vi "configure tdms channels.vi"(4 "samples per channel (1)":u16=1, 6 "type order":T2[](array[typedef]), 8 "error in":errorcluster, 9 "dictionary group names":T1, 10 "dictionary":T1, 11 "tdms file in":refnum<k34>) -> (0 "error out":errorcluster, 3 "tdms file out":refnum<k34>)   [LabVIEW 2015, in "TDMS datalogger runtime.lvclass"]
uses:
  TDMS datalogger runtime.lvclass
  <vilib>/NI/Tag Bus/dictionary/full data dictionary.ctl
  <vilib>/NI/Tag Bus/tag/Data Type.ctl
  <vilib>/NI/Tag Bus/tag/tag descriptor.lvclass
  <vilib>/NI/Tag Bus/dictionary/data dictionary.lvclass
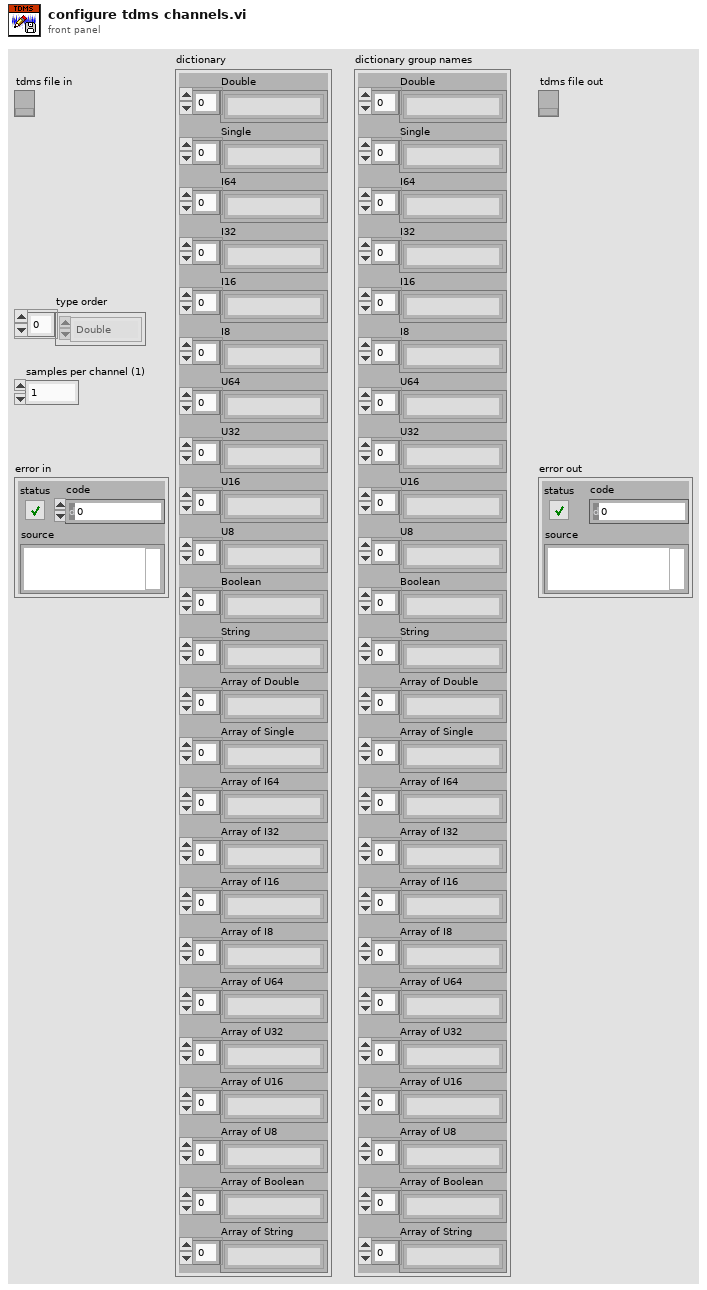
[diagram p1: front panel]
types:
  T1 = typedef "tag bus.lvlib/data dictionary.lvclass/full data dictionary.ctl" = cluster{"Double":string[], "Single":string[], "I64":string[], "I32":string[], "I16":string[], "I8":string[], "U64":string[], "U32":string[], "U16":string[], "U8":string[], "Boolean":string[], "String":string[], "Array of Double":string[], "Array of Single":string[], "Array of I64":string[], "Array of I32":string[], "Array of I16":string[], "Array of I8":string[], "Array of U64":string[], "Array of U32":string[], "Array of U16":string[], "Array of U8":string[], "Array of Boolean":string[], "Array of String":string[]}
  T2 = typedef "tag bus.lvlib/tag descriptor.lvclass/Data Type.ctl" = enum16{"Double", "Single", "I64", "I32", "I16", "I8", "U64", "U32", "U16", "U8", "Boolean", "String", "Array of Double", "Array of Single", "Array of I64", "Array of I32", "Array of I16", "Array of I8", "Array of U64", "Array of U32", "Array of U16", "Array of U8", "Array of Boolean", "Array of String"}
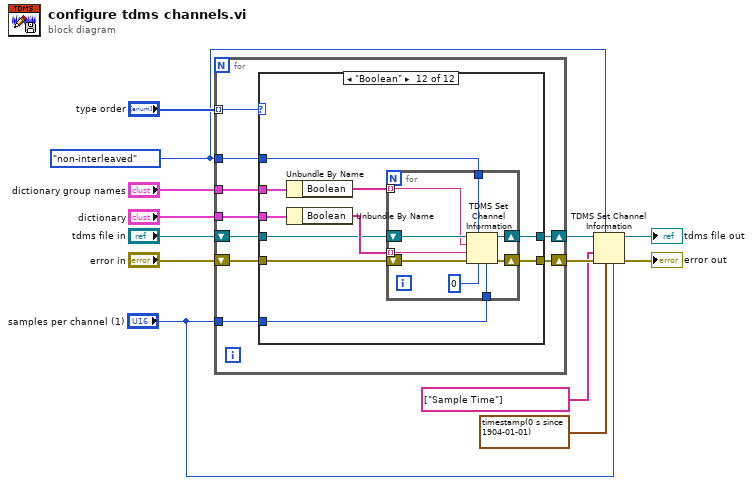
[diagram p0: block diagram]
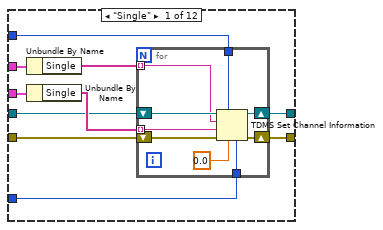
[diagram p2: hidden frame]
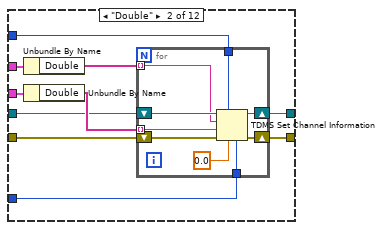
[diagram p3: hidden frame]
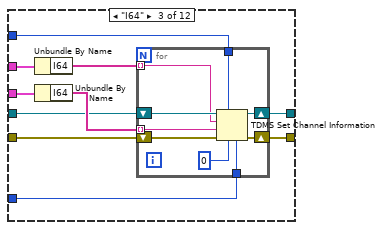
[diagram p4: hidden frame]
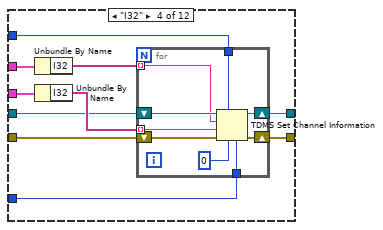
[diagram p5: hidden frame]
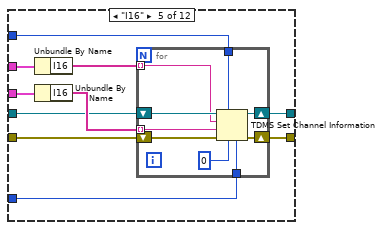
[diagram p6: hidden frame]
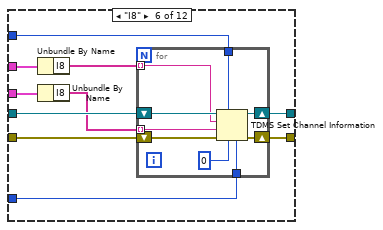
[diagram p7: hidden frame]
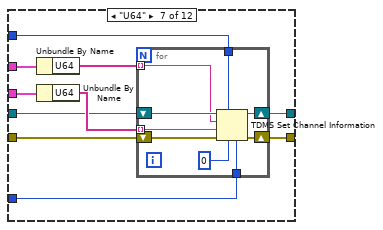
[diagram p8: hidden frame]
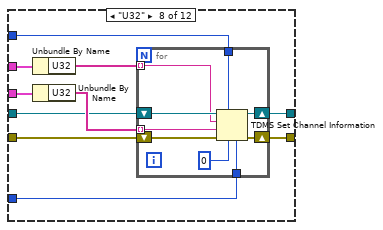
[diagram p9: hidden frame]
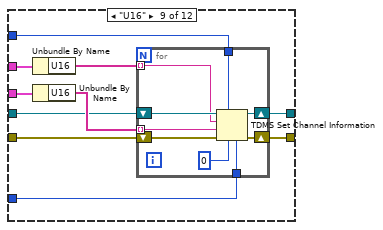
[diagram p10: hidden frame]
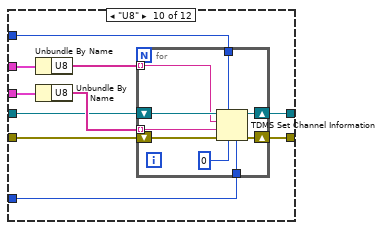
[diagram p11: hidden frame]
diagram:
  w5 = enum16{"non-interleaved", "interleaved"}."non-interleaved" ("data layout (0:non-interleaved)")
  n1 = for {
    tunnel: "dictionary" -> [w15]
    shift-right: [w21] -> w12
    shift-left: "error in" -> [w22]
    shift-right: [w19] -> w7
    shift-left: "tdms file in" -> [w20]
    tunnel: w5 -> [w18]
    tunnel: "samples per channel (1)" -> [w17]
    tunnel: "type order" -> [w16] mode=indexing
    tunnel: "dictionary group names" -> [w14]
    n2 = case shown="\"Boolean\"" w16 {
      tunnel: w22 -> [w27 w42 w66 w80 w100 w127 w138 w162 w180 w199 w214 w220]
      tunnel: [w30 w49 w68 w87 w106 w126 w144 w163 w182 w201 w214 w222] -> w21
      tunnel: w20 -> [w26 w43 w65 w81 w99 w125 w137 w159 w179 w198 w213 w219]
      tunnel: [w29 w47 w61 w85 w104 w124 w139 w156 w175 w194 w213 w215] -> w19
      tunnel: w18 -> [w23 w46 w62 w84 w103 w123 w141 w157 w176 w195 _ w216]
      tunnel: w17 -> [w28 w48 w67 w86 w105 w122 w140 w161 w181 w200 _ w221]
      tunnel: w15 -> [w25 w44 w64 w82 w101 w121 w143 w160 w178 w197 _ w218]
      tunnel: w14 -> [w24 w45 w63 w83 w102 w119 w142 w158 w177 w196 _ w217]
      frame "Single" {
        n3 = Unbundle By Name(w24) -> ("Single"=w31:string[])
        n4 = Unbundle By Name(w25) -> ("Single"=w32:string[])
        n5 = for {
          tunnel: w23 -> [w36]
          tunnel: w28 -> [w35]
          tunnel: w32 -> [w34] mode=indexing
          tunnel: w31 -> [w33] mode=indexing
          shift-right: [w40] -> w30
          shift-left: w27 -> [w41]
          shift-right: [w38] -> w29
          shift-left: w26 -> [w39]
          n6 = TDMS Set Channel Information(4:w35, 6:sgl 0.0, 7:w36, 8:w41, 9:w34, 10:w33, 11:w39) -> (0:w40:errorcluster, 3:w38:refnum<k34>)
        }
      }
      frame "Double" {
        n7 = Unbundle By Name(w45) -> ("Double"=w50:string[])
        n8 = Unbundle By Name(w44) -> ("Double"=w51:string[])
        n9 = for {
          tunnel: w46 -> [w55]
          tunnel: w48 -> [w54]
          tunnel: w51 -> [w53] mode=indexing
          tunnel: w50 -> [w52] mode=indexing
          shift-right: [w59] -> w49
          shift-left: w42 -> [w60]
          shift-right: [w57] -> w47
          shift-left: w43 -> [w58]
          n10 = TDMS Set Channel Information(4:w54, 6:0.0, 7:w55, 8:w60, 9:w53, 10:w52, 11:w58) -> (0:w59:errorcluster, 3:w57:refnum<k34>)
        }
      }
      frame "I64" {
        n11 = Unbundle By Name(w63) -> ("I64"=w69:string[])
        n12 = Unbundle By Name(w64) -> ("I64"=w70:string[])
        n13 = for {
          tunnel: w62 -> [w74]
          tunnel: w67 -> [w73]
          tunnel: w70 -> [w72] mode=indexing
          tunnel: w69 -> [w71] mode=indexing
          shift-right: [w78] -> w68
          shift-left: w66 -> [w79]
          shift-right: [w76] -> w61
          shift-left: w65 -> [w77]
          n14 = TDMS Set Channel Information(4:w73, 6:i64 0, 7:w74, 8:w79, 9:w72, 10:w71, 11:w77) -> (0:w78:errorcluster, 3:w76:refnum<k34>)
        }
      }
      frame "I32" {
        n15 = Unbundle By Name(w83) -> ("I32"=w88:string[])
        n16 = Unbundle By Name(w82) -> ("I32"=w89:string[])
        n17 = for {
          tunnel: w84 -> [w93]
          tunnel: w86 -> [w92]
          tunnel: w89 -> [w91] mode=indexing
          tunnel: w88 -> [w90] mode=indexing
          shift-right: [w97] -> w87
          shift-left: w80 -> [w98]
          shift-right: [w95] -> w85
          shift-left: w81 -> [w96]
          n18 = TDMS Set Channel Information(4:w92, 6:0, 7:w93, 8:w98, 9:w91, 10:w90, 11:w96) -> (0:w97:errorcluster, 3:w95:refnum<k34>)
        }
      }
      frame "I16" {
        n19 = Unbundle By Name(w102) -> ("I16"=w107:string[])
        n20 = Unbundle By Name(w101) -> ("I16"=w108:string[])
        n21 = for {
          tunnel: w103 -> [w112]
          tunnel: w105 -> [w111]
          tunnel: w108 -> [w110] mode=indexing
          tunnel: w107 -> [w109] mode=indexing
          shift-right: [w116] -> w106
          shift-left: w100 -> [w117]
          shift-right: [w114] -> w104
          shift-left: w99 -> [w115]
          n22 = TDMS Set Channel Information(4:w111, 6:i16 0, 7:w112, 8:w117, 9:w110, 10:w109, 11:w115) -> (0:w116:errorcluster, 3:w114:refnum<k34>)
        }
      }
      frame "I8" {
        n23 = Unbundle By Name(w119) -> ("I8"=w118:string[])
        n24 = Unbundle By Name(w121) -> ("I8"=w120:string[])
        n25 = for {
          tunnel: w123 -> [w131]
          tunnel: w122 -> [w130]
          tunnel: w120 -> [w129] mode=indexing
          tunnel: w118 -> [w128] mode=indexing
          shift-right: [w135] -> w126
          shift-left: w127 -> [w136]
          shift-right: [w133] -> w124
          shift-left: w125 -> [w134]
          n26 = TDMS Set Channel Information(4:w130, 6:i8 0, 7:w131, 8:w136, 9:w129, 10:w128, 11:w134) -> (0:w135:errorcluster, 3:w133:refnum<k34>)
        }
      }
      frame "U64" {
        n27 = Unbundle By Name(w142) -> ("U64"=w145:string[])
        n28 = Unbundle By Name(w143) -> ("U64"=w146:string[])
        n29 = for {
          tunnel: w141 -> [w150]
          tunnel: w140 -> [w149]
          tunnel: w146 -> [w148] mode=indexing
          tunnel: w145 -> [w147] mode=indexing
          shift-right: [w154] -> w144
          shift-left: w138 -> [w155]
          shift-right: [w152] -> w139
          shift-left: w137 -> [w153]
          n30 = TDMS Set Channel Information(4:w149, 6:u64 0, 7:w150, 8:w155, 9:w148, 10:w147, 11:w153) -> (0:w154:errorcluster, 3:w152:refnum<k34>)
        }
      }
      frame "U32" {
        n31 = Unbundle By Name(w158) -> ("U32"=w164:string[])
        n32 = Unbundle By Name(w160) -> ("U32"=w165:string[])
        n33 = for {
          tunnel: w157 -> [w169]
          tunnel: w161 -> [w168]
          tunnel: w165 -> [w167] mode=indexing
          tunnel: w164 -> [w166] mode=indexing
          shift-right: [w173] -> w163
          shift-left: w162 -> [w174]
          shift-right: [w171] -> w156
          shift-left: w159 -> [w172]
          n34 = TDMS Set Channel Information(4:w168, 6:u32 0, 7:w169, 8:w174, 9:w167, 10:w166, 11:w172) -> (0:w173:errorcluster, 3:w171:refnum<k34>)
        }
      }
      frame "U16" {
        n35 = Unbundle By Name(w177) -> ("U16"=w183:string[])
        n36 = Unbundle By Name(w178) -> ("U16"=w184:string[])
        n37 = for {
          tunnel: w176 -> [w188]
          tunnel: w181 -> [w187]
          tunnel: w184 -> [w186] mode=indexing
          tunnel: w183 -> [w185] mode=indexing
          shift-right: [w192] -> w182
          shift-left: w180 -> [w193]
          shift-right: [w190] -> w175
          shift-left: w179 -> [w191]
          n38 = TDMS Set Channel Information(4:w187, 6:u16 0, 7:w188, 8:w193, 9:w186, 10:w185, 11:w191) -> (0:w192:errorcluster, 3:w190:refnum<k34>)
        }
      }
      frame "U8" {
        n39 = Unbundle By Name(w196) -> ("U8"=w202:string[])
        n40 = Unbundle By Name(w197) -> ("U8"=w203:string[])
        n41 = for {
          tunnel: w195 -> [w207]
          tunnel: w200 -> [w206]
          tunnel: w203 -> [w205] mode=indexing
          tunnel: w202 -> [w204] mode=indexing
          shift-right: [w211] -> w201
          shift-left: w199 -> [w212]
          shift-right: [w209] -> w194
          shift-left: w198 -> [w210]
          n42 = TDMS Set Channel Information(4:w206, 6:u8 0, 7:w207, 8:w212, 9:w205, 10:w204, 11:w210) -> (0:w211:errorcluster, 3:w209:refnum<k34>)
        }
      }
      frame Default {
      }
      frame "Boolean" {
        n43 = Unbundle By Name(w217) -> ("Boolean"=w223:string[])
        n44 = Unbundle By Name(w218) -> ("Boolean"=w224:string[])
        n45 = for {
          tunnel: w216 -> [w228]
          tunnel: w221 -> [w227]
          tunnel: w224 -> [w226] mode=indexing
          tunnel: w223 -> [w225] mode=indexing
          shift-right: [w232] -> w222
          shift-left: w220 -> [w233]
          shift-right: [w230] -> w215
          shift-left: w219 -> [w231]
          n46 = TDMS Set Channel Information(4:w227, 6:i8 0, 7:w228, 8:w233, 9:w226, 10:w225, 11:w231) -> (0:w232:errorcluster, 3:w230:refnum<k34>)
        }
      }
    }
  }
  n47 = TDMS Set Channel Information(4:"samples per channel (1)", 6:timestamp(0 s since 1904-01-01), 7:w5, 8:w12, 9:string[] ["Sample Time"] ("channel name(s)"), 11:w7) -> (0:→"error out":errorcluster, 3:→"tdms file out":refnum<k34>)  [unwired: 1 in]
